vi "Read Sensor Data.vi"(8 "error in (no error)":errorcluster, 10 "Channel (1:1)":u16(ring)=1 items=["1"=1, "2"=2, "3"=3, "4"=4, "5"=5, "6"=6, "7"=7, "8"=8, "9"=9, "10"=10, "11"=11, "12"=12, "13"=13, "14"=14, "15"=15, "16"=16, "A (Control Input)"=17], 11 "VISA resource name":refnum<visa-resource-name>) -> (0 "error out":errorcluster, 1 "Kelvin Reading":dbl min=0.0 max=1000.0 step=1e-05 format="%^.5e", 2 "Resistance Reading":dbl min=0.0 max=63200000.0 step=1e-05 format="%^.5e", 3 "VISA resource name out":refnum<visa-resource-name>, 4 "Power Reading":dbl min=0.0 max=0.01 step=1e-05 format="%^.5e", 5 "Quadrature Reading":dbl min=0.0 max=0.01 step=1e-05 format="%^.5e")   [LabVIEW 2018, in "Lake Shore 372.lvlib"]
doc: "Queries the instrument for a channel's sensor reading in Resistance, Quadrature, Kelvin, and Power. This VI uses the <B>SRDG?</B>, <B>KRDG?</B>, <B>RDGPWR?</B>, and <B>QRDG?</B> commands. Please refer to Model 372 manual for further explanation."
uses:
  Lake Shore 372.lvlib
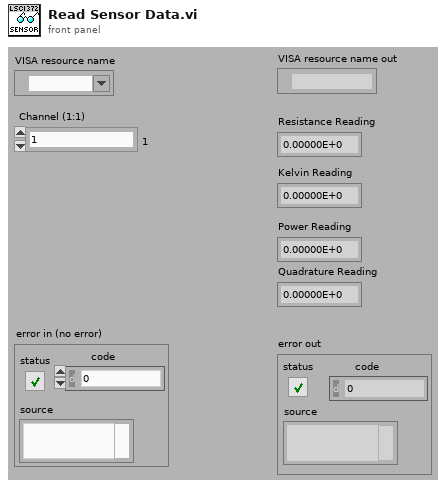
[diagram p1: front panel]
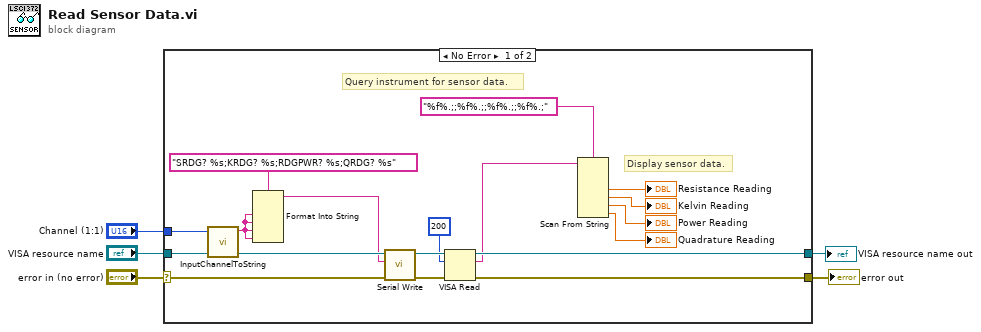
[diagram p0: block diagram]
diagram:
  n1 = case shown="No Error" "error in (no error)" {
    selector: "error in (no error)" -> [w7 w23]
    tunnel: [w22 w23] -> w5
    tunnel: [w21 w24] -> w4
    tunnel: "Channel (1:1)" -> [w20 _]
    tunnel: "VISA resource name" -> [w11 w24]
    frame No Error {
      # "Display sensor data."
      # "Query instrument for sensor data."
      n2 = call "InputChannelToString.vi"("Channel (1)"=w20) -> ("Channel Str"=w13:string)  [unwired: 10 in]
      n3 = Format Into String(format string="SRDG? %s;KRDG? %s;RDGPWR? %s;QRDG? %s", w13, w13, w13, w13) -> (resulting string=w10:string)  [unwired: 2 in, 1 out]
      n4 = call "Serial Write.vi"("error in (no error)"=w7, "Write Buffer (\"\")"=w10, "VISA resource name"=w11) -> ("error out"=w12:errorcluster, "VISA resource name out"=w9:refnum<visa-resource-name>)  [unwired: 6 in, 1 out]
      n5 = VISA Read(VISA resource name=w9, byte count=200, error in (no error)=w12) -> (VISA resource name out=w21:refnum<visa-resource-name>, read buffer=w6:string, error out=w22:errorcluster)  [unwired: 1 out]
      n6 = Scan From String(format string="%f%.;;%f%.;;%f%.;;%f%.;", input string=w6) -> (output 1=→"Resistance Reading":dbl, output 2=→"Kelvin Reading":dbl, output 3=→"Power Reading":dbl, output 4=→"Quadrature Reading":dbl)  [unwired: 6 in, 3 out]
    }
    frame Error {
    }
  }
  "VISA resource name out" <- w4
  "error out" <- w5
